vi "analyze.vi"(1 "classes per student":i32, 2 "rearranged Student data":i32[][](array[numeric])) -> (0 "Array":i32[](array[numeric]))   [LabVIEW 2009]
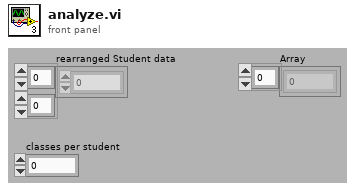
[diagram p1: front panel]
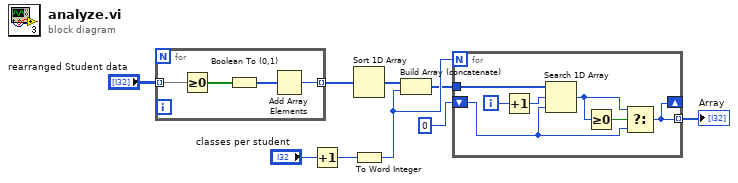
[diagram p0: block diagram]
diagram:
  n1 = for {
    tunnel: "rearranged Student data" -> [w13] mode=indexing
    tunnel: [w10] -> w2 mode=indexing
    n2 = Greater Or Equal To 0?(x=w13) -> (x >= 0?=w12:bool[])
    n3 = Boolean To (0,1)(Boolean=w12) -> (0, 1=w11:i16[])
    n4 = Add Array Elements(numeric array=w11) -> (sum=w10:i16)
  }
  n5 = Increment(x="classes per student") -> (x+1=w5:i32)
  n6 = Sort 1D Array(array=w2) -> (sorted array=w3:i16[])
  n7 = To Word Integer(number=w5) -> (16bit integer=w8:i16)
  n8 = Build Array (concatenate)(w3, w8) -> (w6:i16[])
  n9 = for {
    N: w8 -> [_]
    tunnel: w6 -> [w20]
    shift-right: [w14] -> _
    shift-left: 0 ("index of element") -> [w17]
    tunnel: [w14] -> w9 mode=indexing
    i -> [w19]
    n10 = Increment(x=w19) -> (x+1=w18:i32)
    n11 = Search 1D Array(1D array=w20, element=w18, start index (0)=w17) -> (index of element=w16:i32)
    n12 = Greater Or Equal To 0?(x=w16) -> (x >= 0?=w15:bool)
    n13 = Select(t=w16, s=w15, f=w17) -> (s? t:f=w14:i32)
  }
  "Array" <- w9
